vi "Timer_New.vi"() -> (3 "TIMER":T1 {"Accumulated TIme" format="%13.5p"; "StartTime" format="%13.5p"})   [LabVIEW 2019, in "Trajectory_Library.lvlib"]
doc: "Creates and initializes a Timer data cluster.\n\nOutputs:\n - Timer -- The initialized Timer data cluster"
uses:
  Trajectory_Library.lvlib
  TIMER.ctl
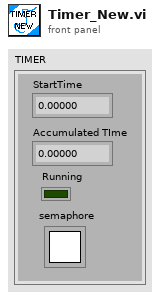
[diagram p1: front panel]
types:
  T1 = typedef "Trajectory_Library.lvlib/TIMER.ctl" = cluster{"StartTime":dbl, "Accumulated TIme":dbl, "Running":bool, "semaphore":T2}
  T2 = typedef "Semaphore RefNum" = refnum<k1>
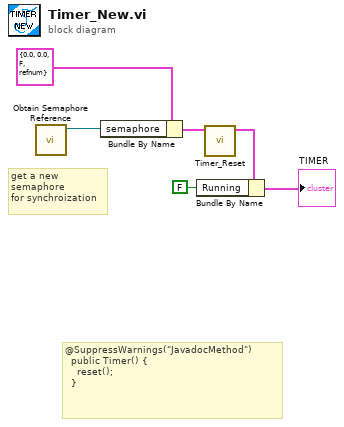
[diagram p0: block diagram]
diagram:
  # "get a new \nsemaphore\nfor synchroization"
  # "@SuppressWarnings(\"JavadocMethod\")\n  public Timer() {\n    reset();\n  }"
  n1 = call <vilib>:"Obtain Semaphore Reference.vi"() -> ("semaphore"=w1:T2)  [unwired: 5 in, 2 out]
  n2 = Bundle By Name(cluster=T1 {"StartTime"=0.0, "Accumulated TIme"=0.0, "Running"=FALSE, "semaphore"=refnum} ("in TIMER"), "semaphore"=w1) -> (w2:T1)
  n3 = call "Timer_Reset.vi"("in TIMER"=w2) -> ("out TIMER"=w6:T1)  [unwired: 10 in]
  n4 = Bundle By Name(cluster=w6, "Running"=FALSE) -> (→"TIMER":T1)
